vi "USBCam.vi"() -> ()   [LabVIEW 2014]
doc: "This is the main user interface of the Raman spectroscopy system."
uses:
  TypeDef/States.ctl
  <vilib>/Utility/miscctls.llb/LVPoint32TypeDef.ctl
  TypeDef/LaserSpot.ctl
panel:
  out "Spot Y":dbl
  out "Spot X":dbl
  in  "Box":cluster{"Width":dbl, " Height":dbl}={"Width"=200.0, " Height"=214.0}
  in  "Down":bool
  in  "Top":bool
  in  "Right":bool
  in  "Left":bool
  in  "Snap":bool
  out "Boolean":bool
  in  "LaserSpot":bool
  out "Initialization finished":bool
  out "ZoomRatio":dbl format="%#_2g"
  out "Live video":picture caption="600 x 480"
  in  "Camera ID":u32
  out "Bits/Pixel":i32=8
  in  "Autogain":bool
  in  "Master Gain":i32(slide) min=0 max=100 scale=0.0..100.0
  in  "Hotpixel correction 2":bool
  in  "Blacklevel compensation":bool
  in  "Edge Filter":i32(ring)=2 items=["High"=1, "Low"=2]
  in  "Edge Filter Enable / Disable":bool
  in  "Exposure time (ms)":dbl(slide)=100.65900000000002 min=0.06675 max=71.556 step=0.06675 scale=0.06675..71.556 scale format="%#.3g"
  in  "Pixel clock":i32(slide)=20 min=5 max=43 scale=5.0..43.0
  in  "Frame rate":dbl(slide)=9.827169720568149 min=4.876716604244694 max=13.962044182888818 step=6.675e-05 scale=4.876716604244694..13.962044182888818 scale format="%^#_3g"
  in  "Blacklevel Offset":i32(slide) min=0 max=255 scale=0.0..255.0
  out "FPS":dbl=6.258409738085552
  out "Width":i32=640
  out "Height":i32=480
  in  "Quit":bool
  # "Camera Control"
  # "Objective: CFI Plan Fluor ELWD 60x (1.27 NA) \nThe depth of field: 1.78 um\nPixel Size: 0.0877um/px"
  # "Adjust laser spot lightly"
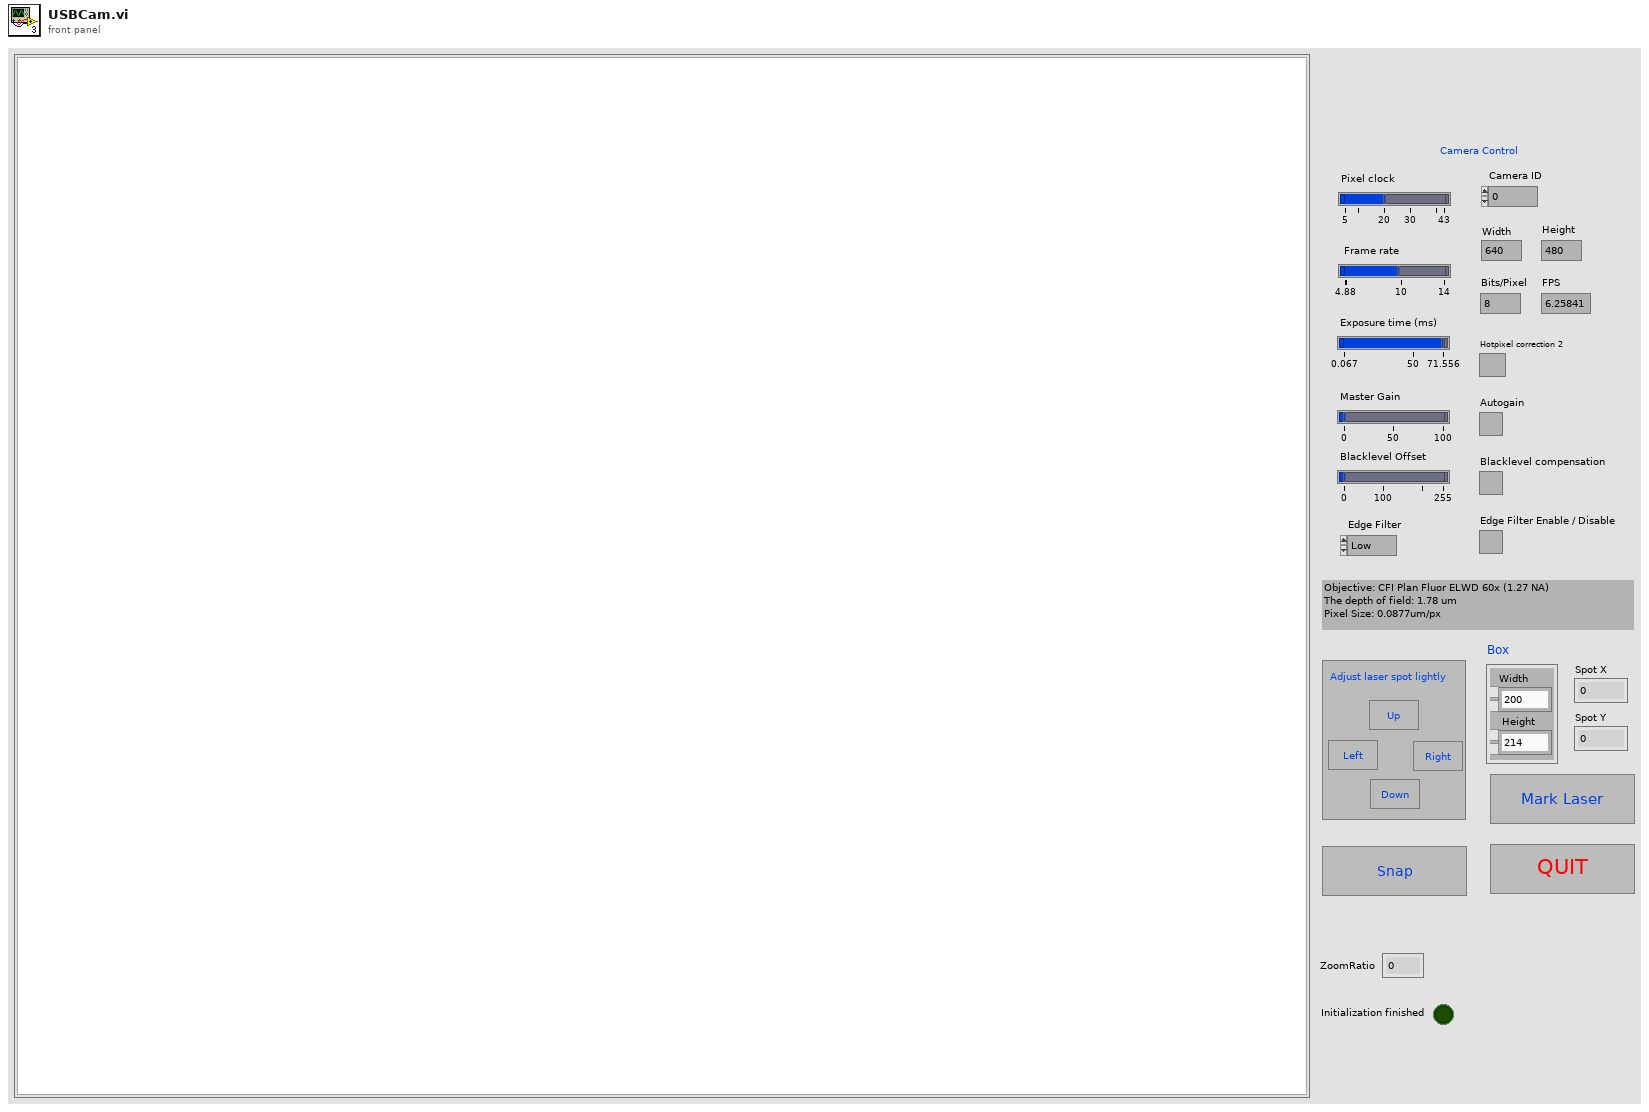
[diagram p1: front panel]
types:
  T1 = typedef "LaserSpot.ctl" = cluster{"Laser X":dbl, "Laser Y":dbl}
  T2 = cluster{"left":i16, "top":i16, "right":i16, "bottom":i16}
  T3 = typedef "LVPoint32TypeDef.ctl" = cluster{"Horizontal":i32, "Vertical":i32}
  T4 = typedef "States.ctl" = enum16{"Initialize", "CMOS live", "Shut down"}
  T5 = cluster{"Width":u16, "Style":enum32{"Solid", "Dash", "Dot", "DashDot", "DashDotDot"}}
  T6 = typedef "LVBoundsTypeDef.ctl" = cluster{"Width":u32, "Height":u32}
  T7 = typedef "imagedata.ctl" = cluster{"image type":i32, "image depth":i32, "image":u8[], "mask":u8[], "colors":u32[], "Rectangle":cluster{"left":i16, "top":i16, "right":i16, "bottom":i16}}
  T8 = typedef "LVPositionTypeDef.ctl" = cluster{"Left":i32, "Top":i32}
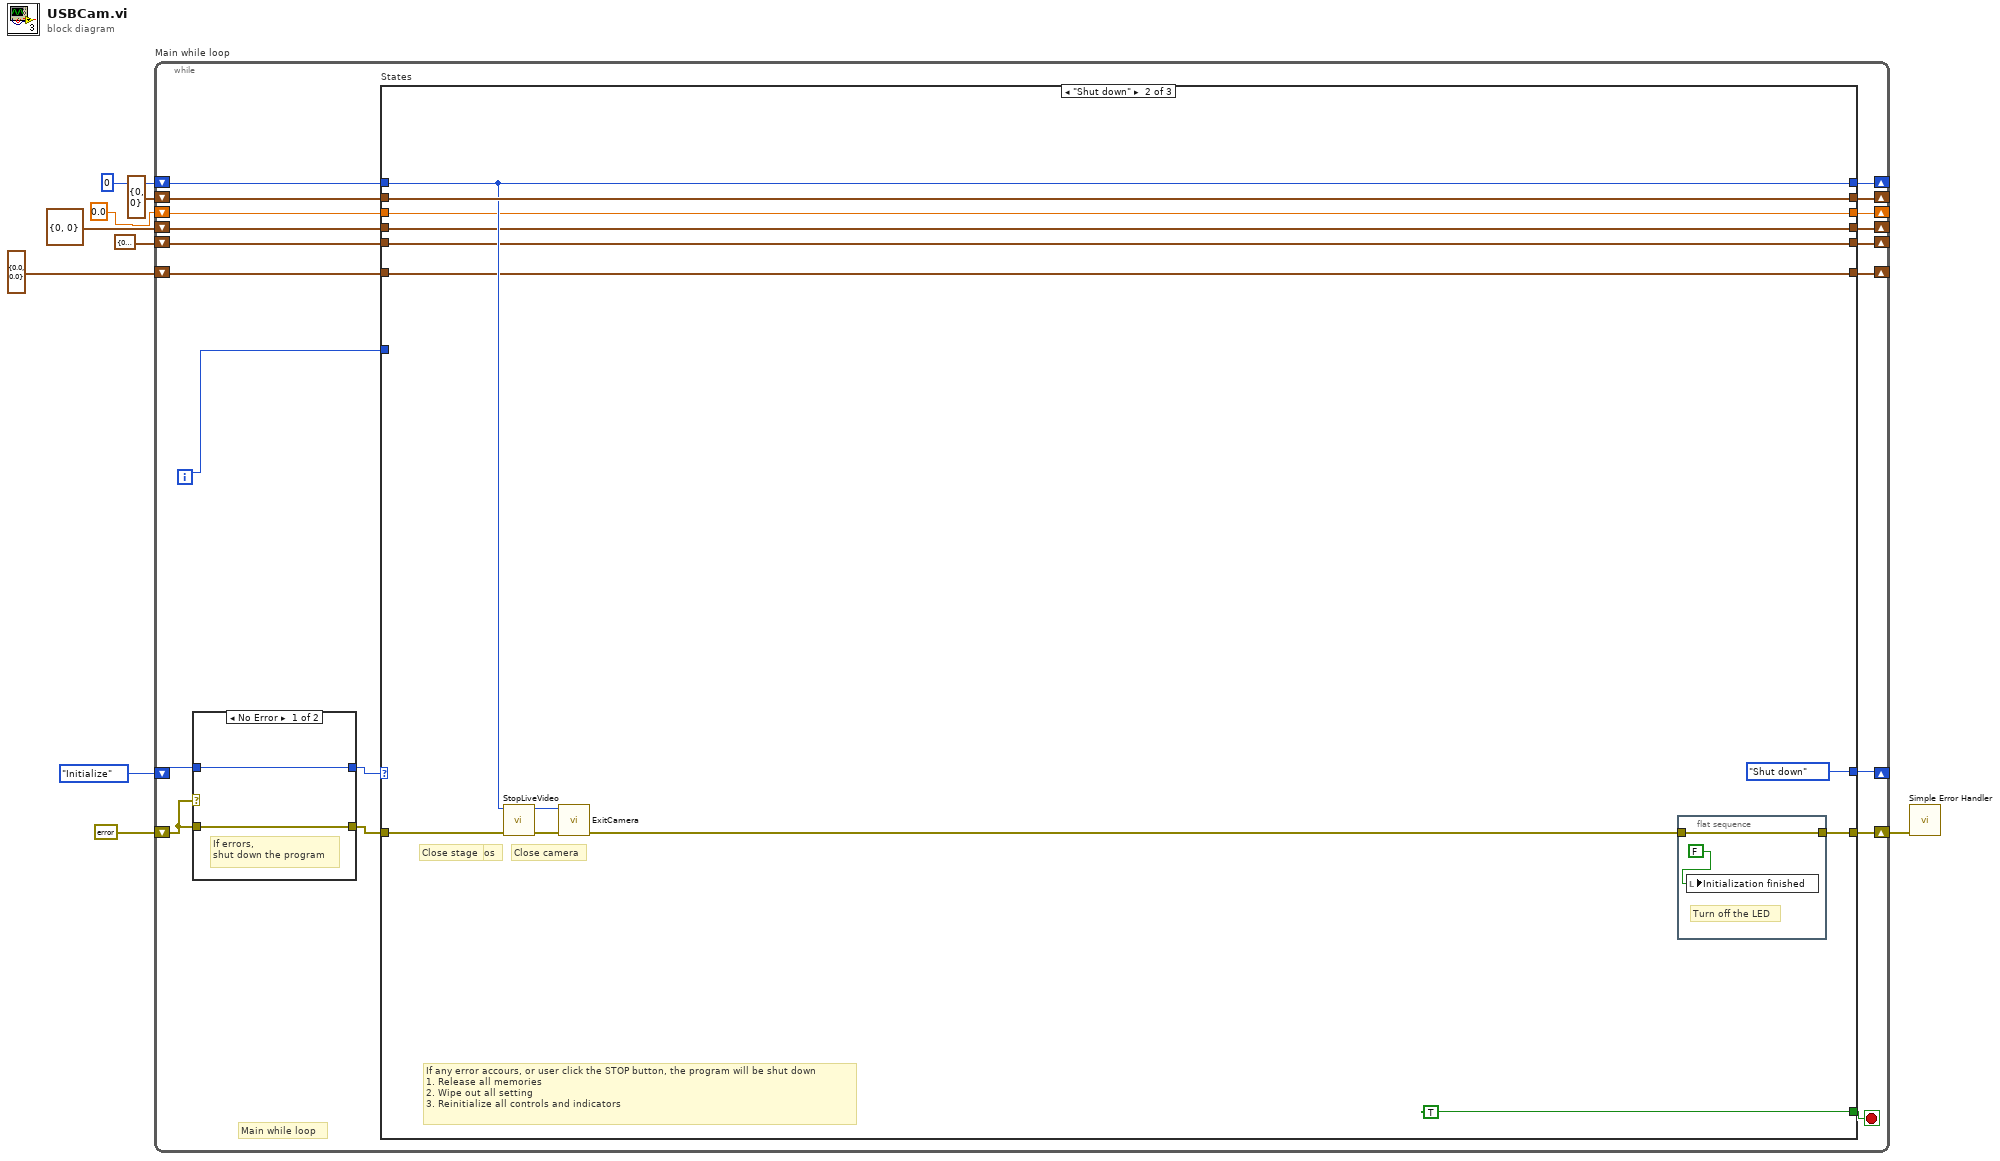
[diagram p0: block diagram]
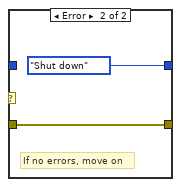
[diagram p2: hidden frame]
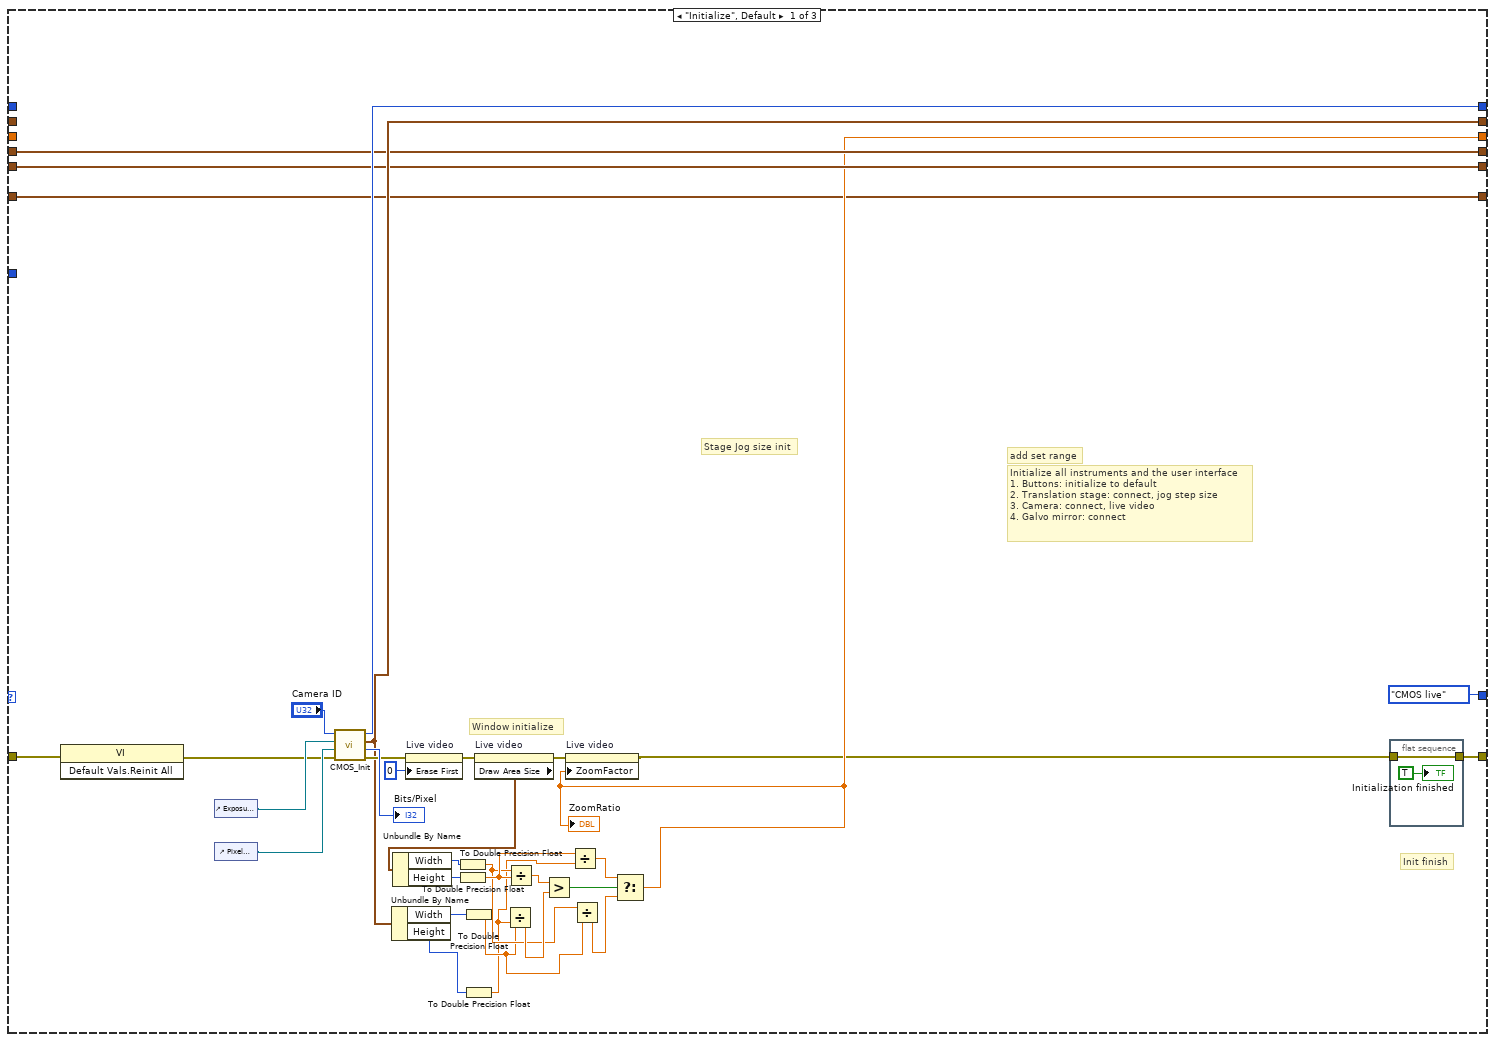
[diagram p3: hidden frame]
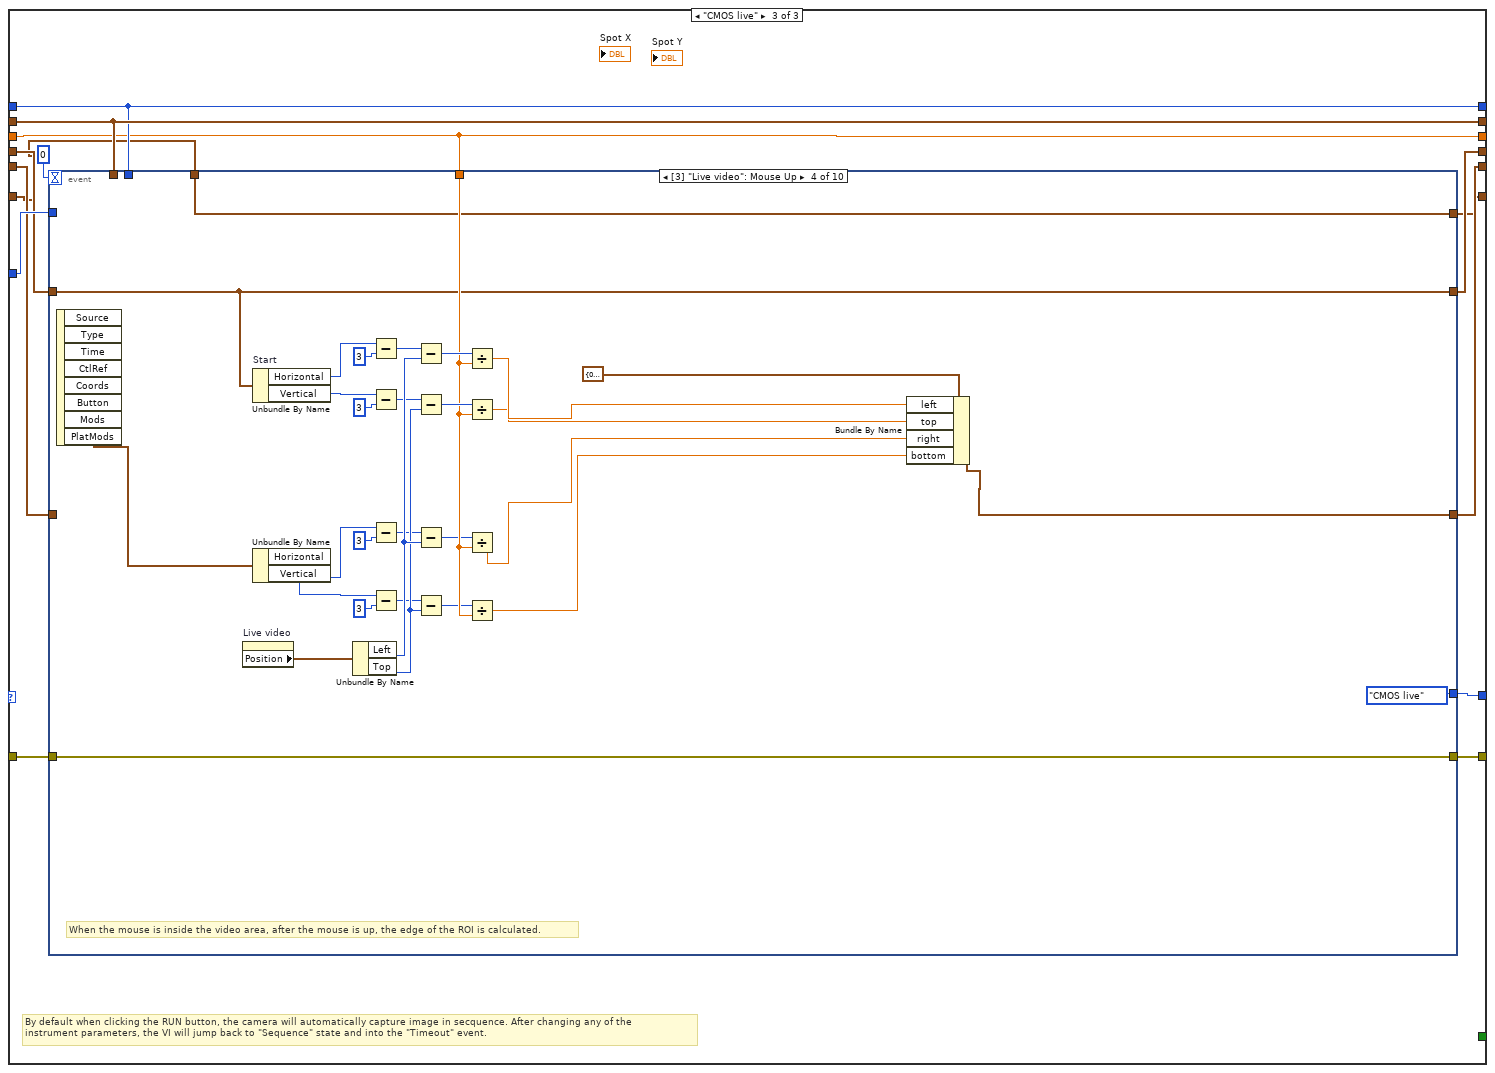
[diagram p4: hidden frame]
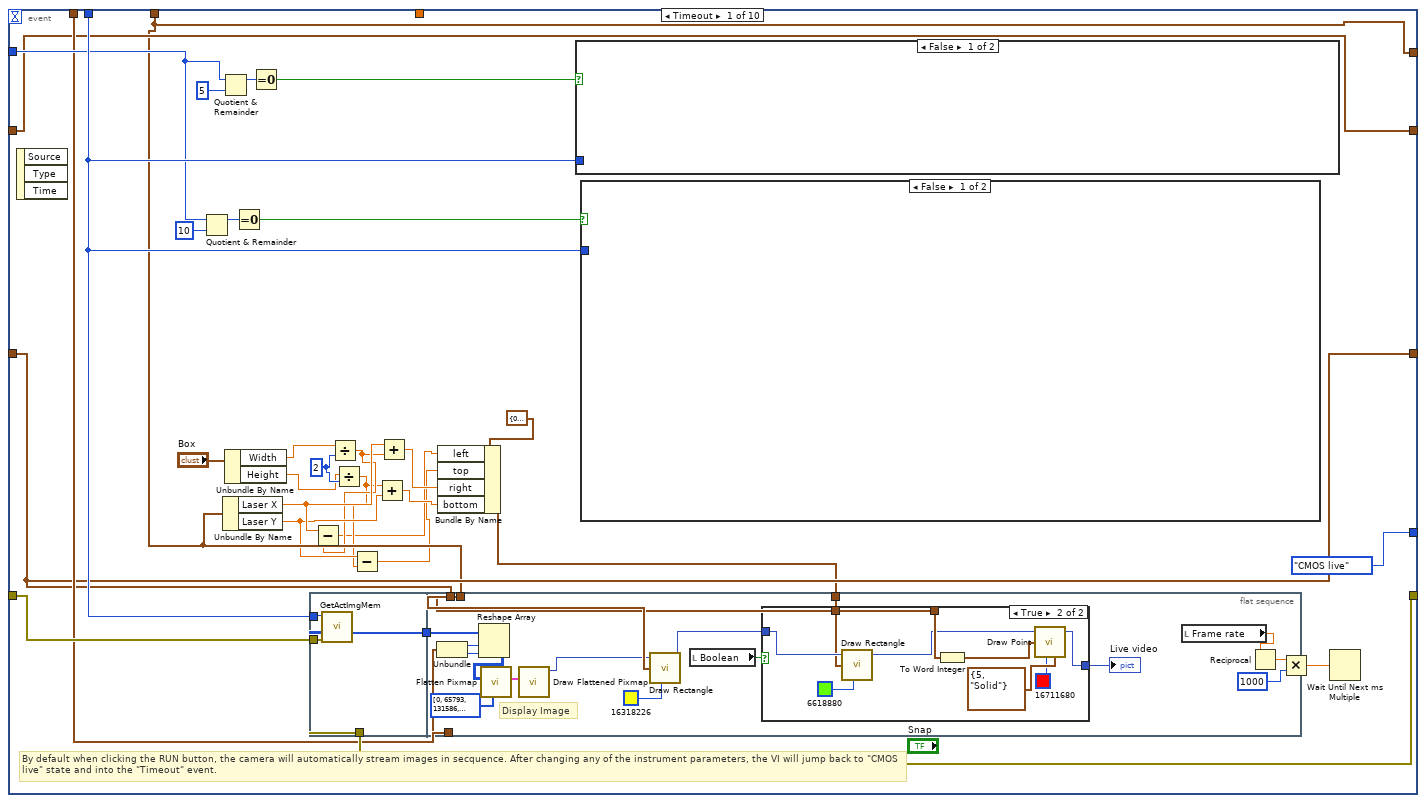
[diagram p5: hidden frame]
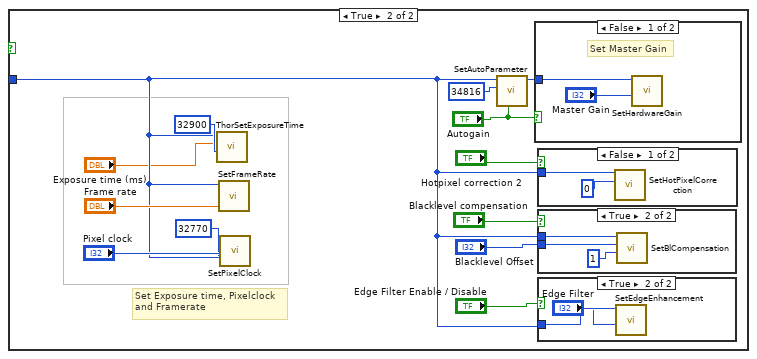
[diagram p6: hidden frame]
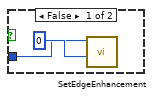
[diagram p7: hidden frame]
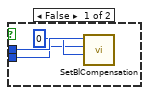
[diagram p8: hidden frame]
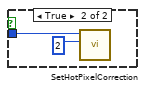
[diagram p9: hidden frame]
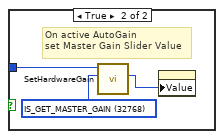
[diagram p10: hidden frame]
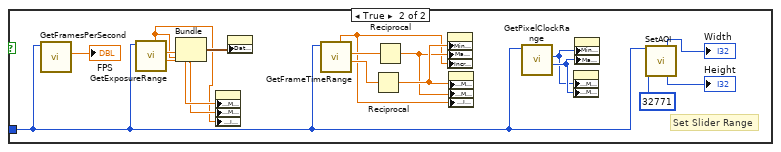
[diagram p11: hidden frame]
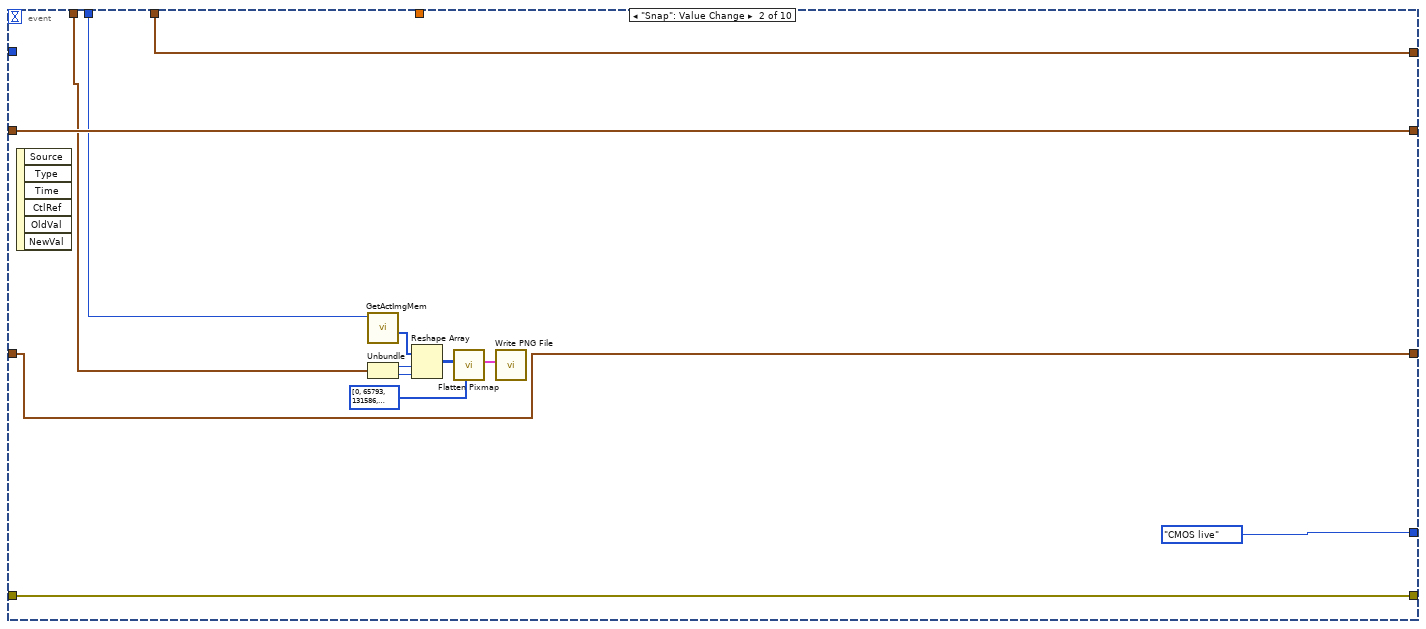
[diagram p13: hidden frame]
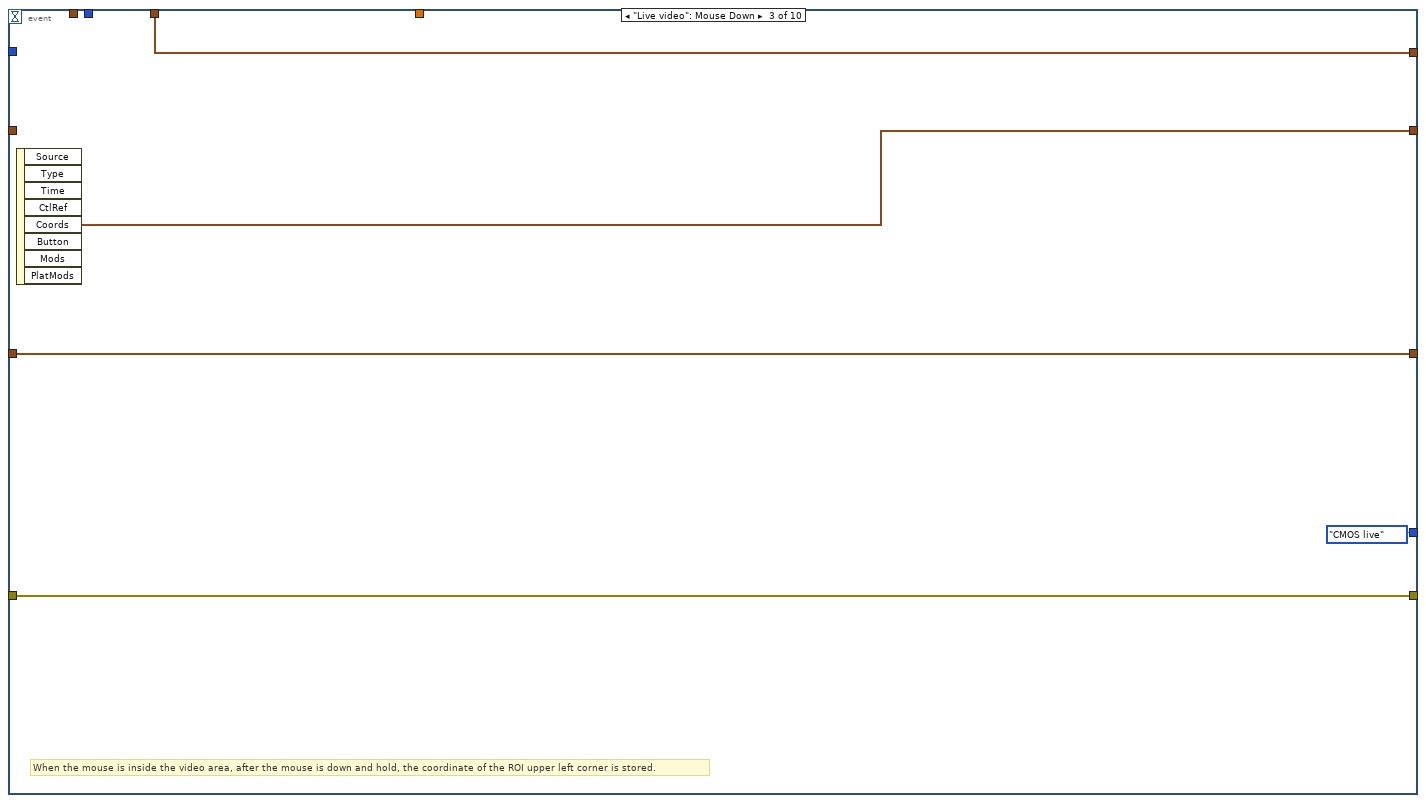
[diagram p14: hidden frame]
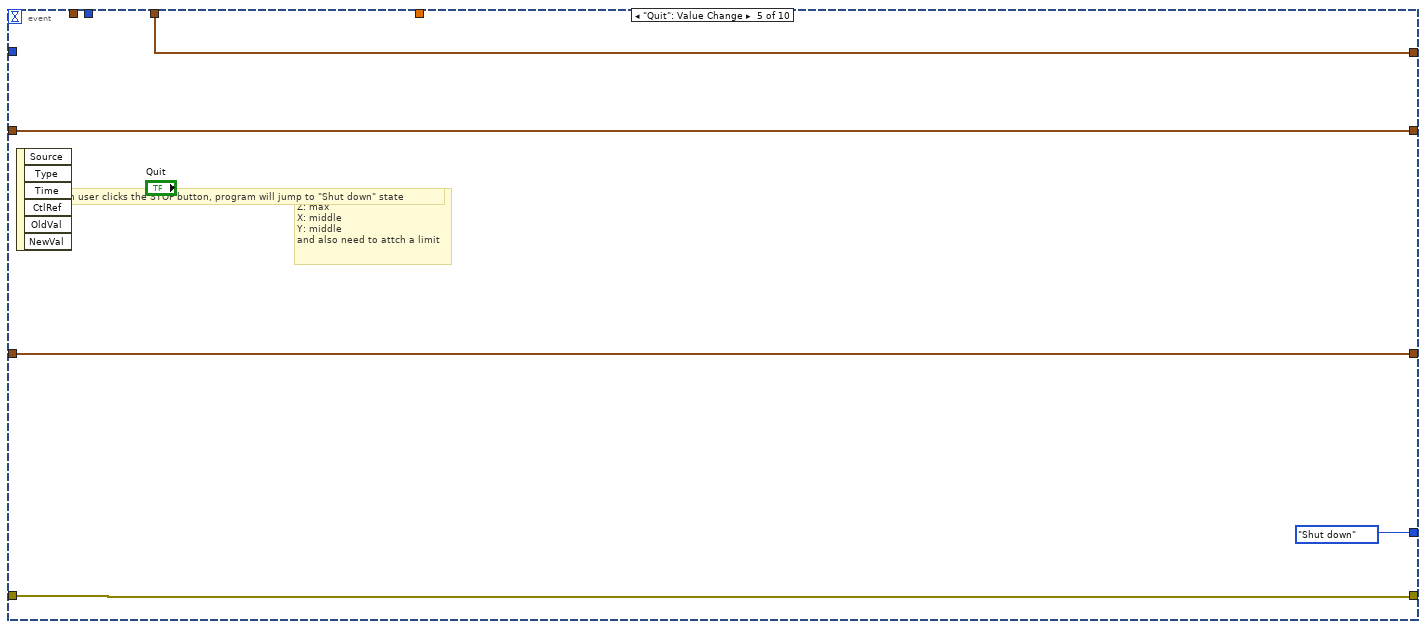
[diagram p15: hidden frame]
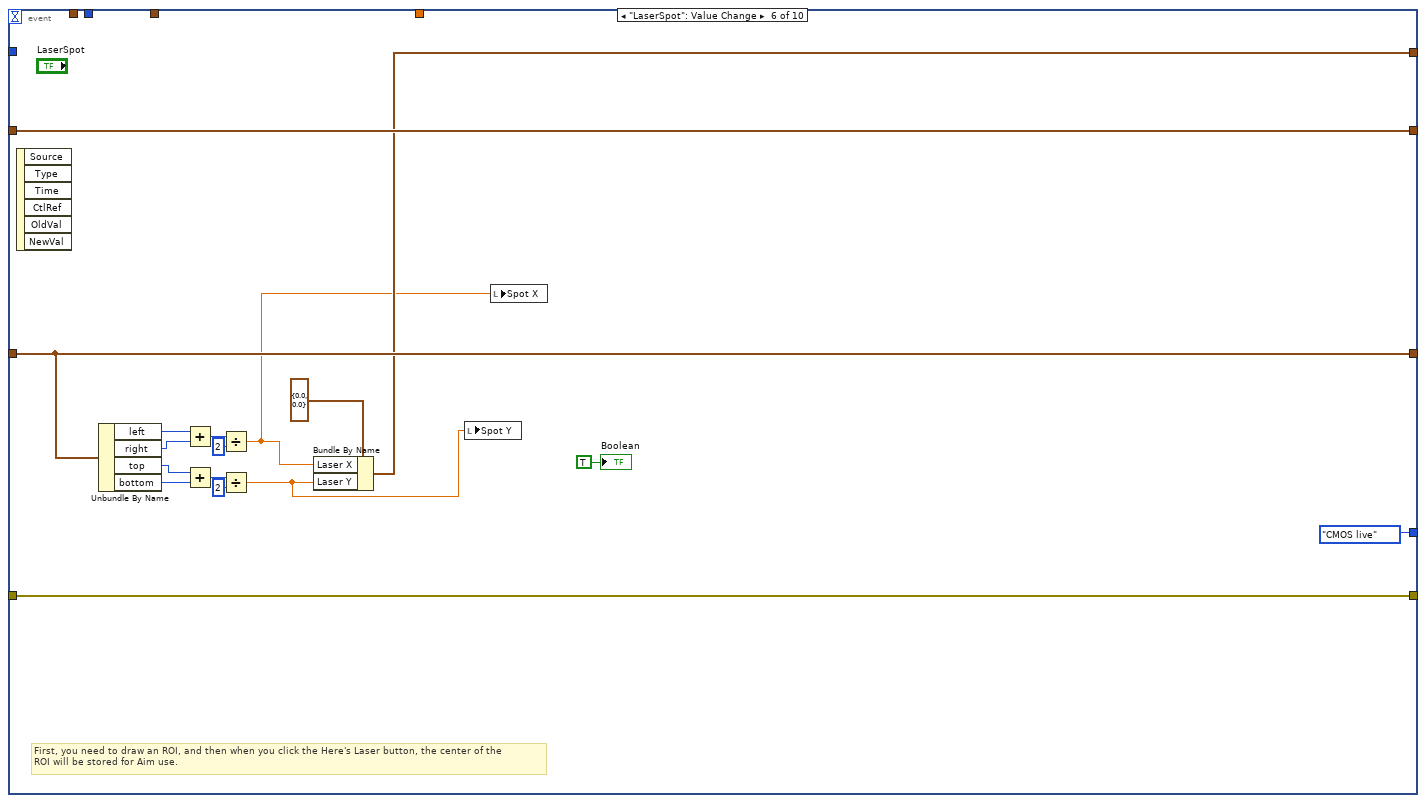
[diagram p16: hidden frame]
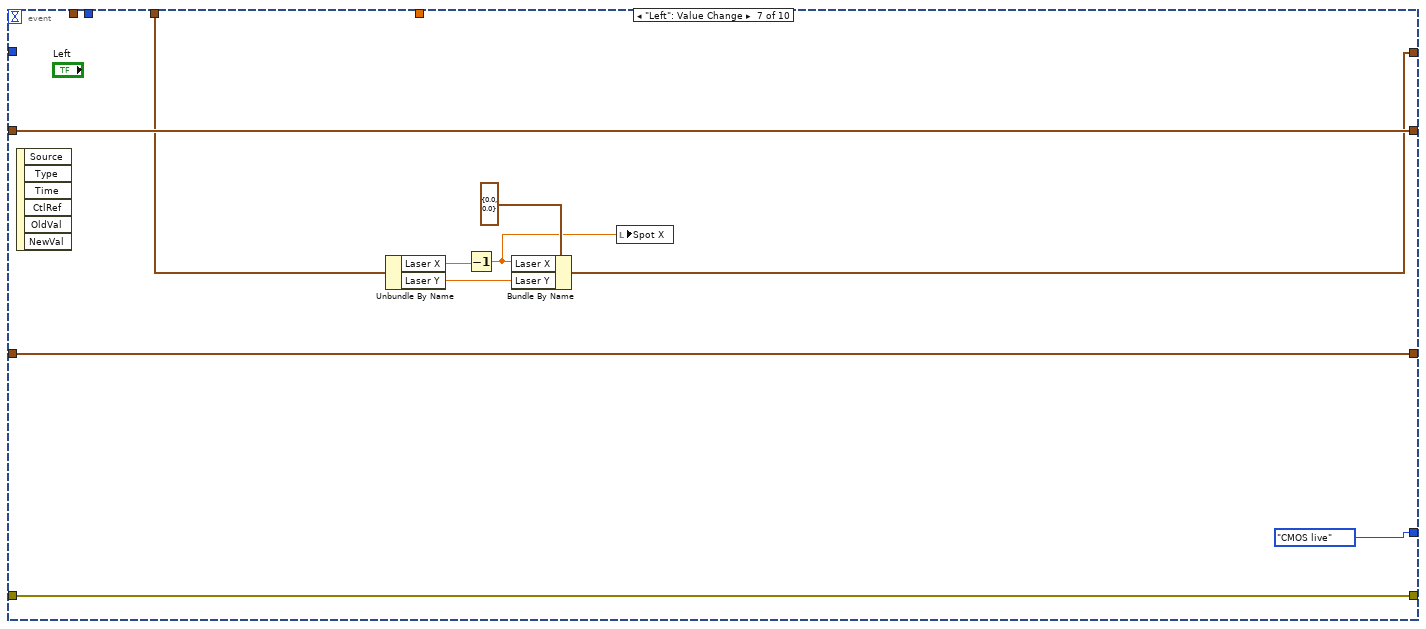
[diagram p17: hidden frame]
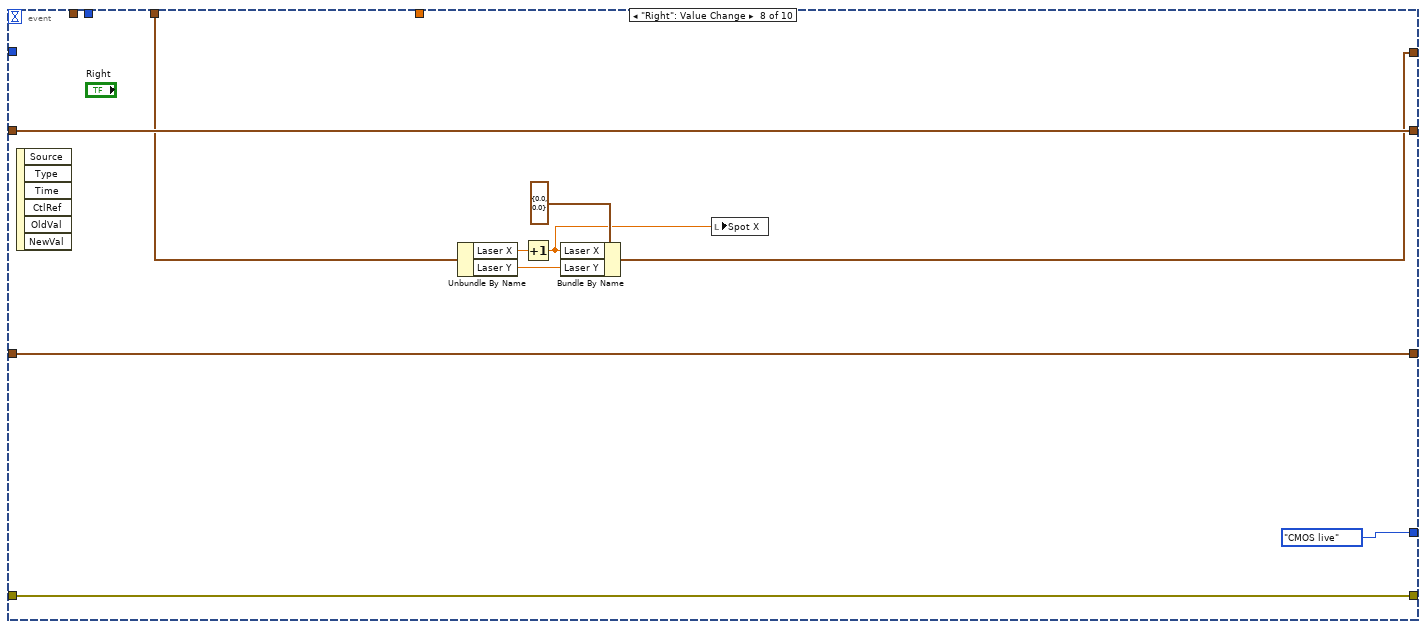
[diagram p18: hidden frame]
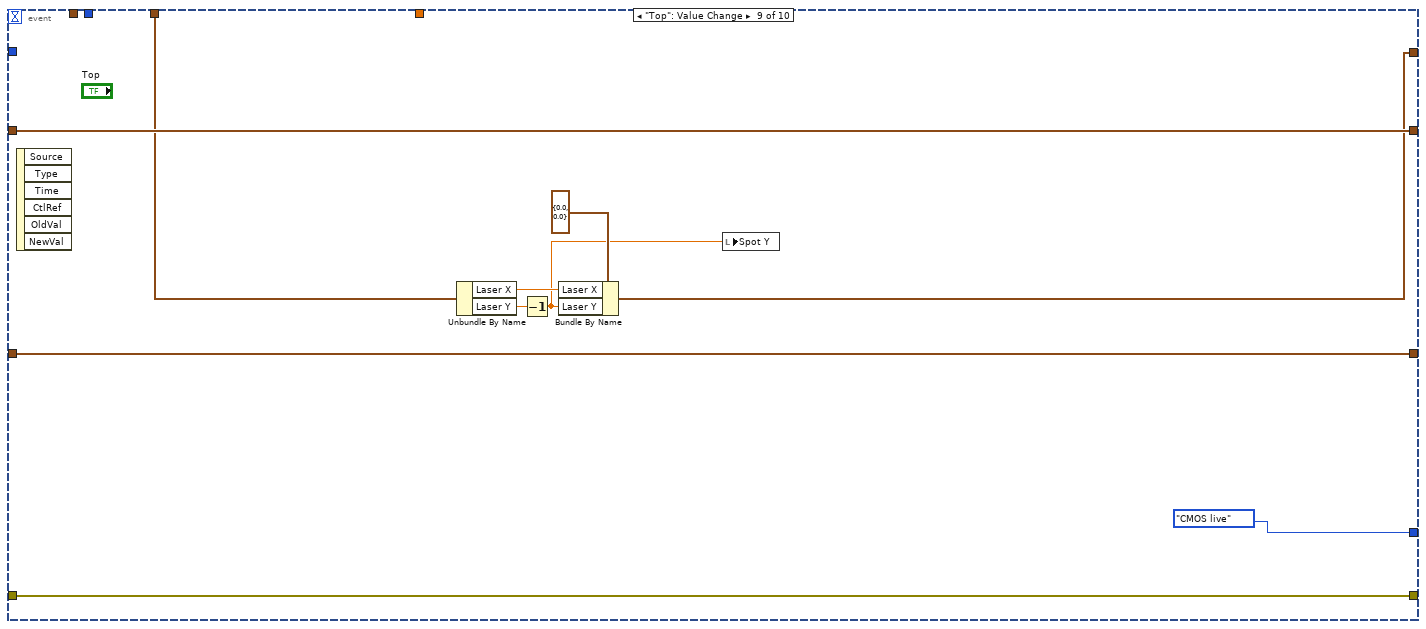
[diagram p19: hidden frame]
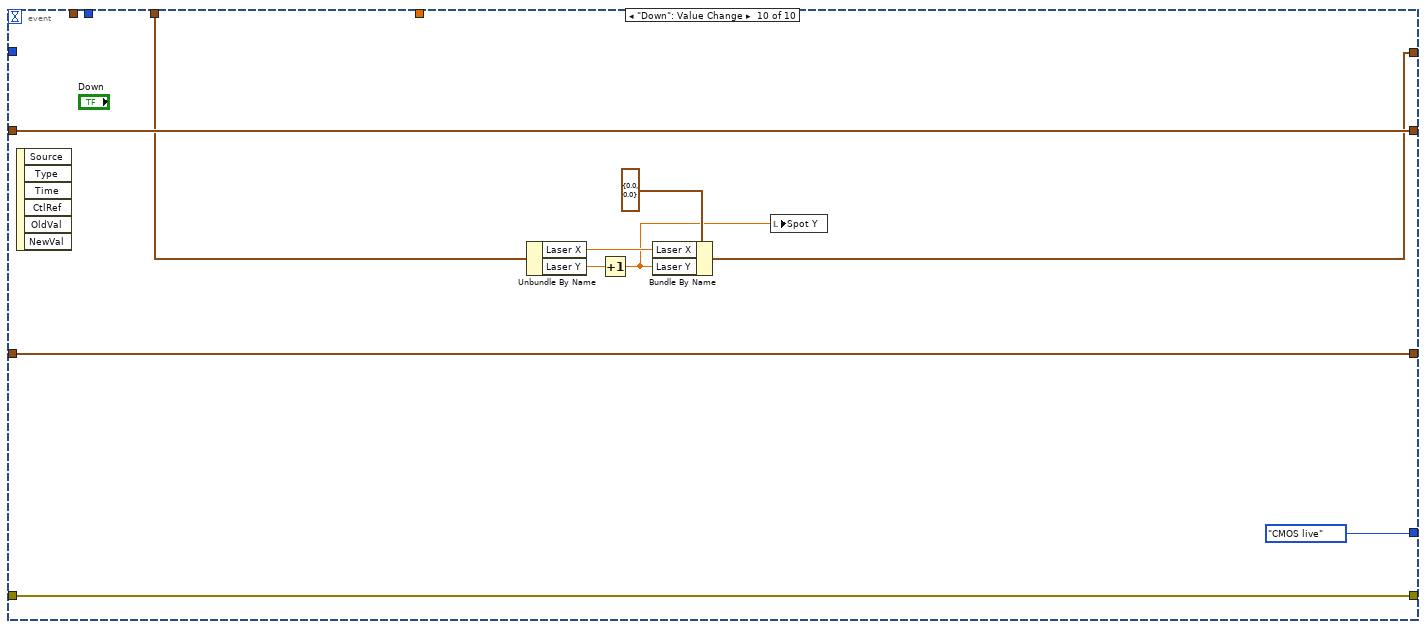
[diagram p20: hidden frame]
diagram:
  n1 = while "Main while loop" {
    shift-right: [w24] -> _
    shift-left: States."Initialize" -> [w29]
    shift-right: [w27] -> w7
    shift-left: errorcluster {"status"=FALSE, "code"=0, "source"=""} ("error out") -> [w23]
    shift-right: [w22] -> _
    shift-left: u32 0 ("CMOS Handle Out") -> [w21]
    shift-right: [w19] -> _
    shift-left: cluster{"Height":i32, "Width":i32} {"Height"=0, "Width"=0} ("WidthAndHeight") -> [w18]
    shift-right: [w17] -> _
    shift-left: 0.0 -> [w12]
    shift-right: [w16] -> _
    shift-left: T3 {"Horizontal"=0, "Vertical"=0} ("Coords") -> [w15]
    shift-right: [w14] -> _
    shift-left: T2 {"left"=0, "top"=0, "right"=0, "bottom"=0} ("rect") -> [w13]
    shift-right: [w11] -> _
    shift-left: T1 {"Laser X"=0.0, "Laser Y"=0.0} ("LaserSpot 2") -> [w10]
    i -> [w20]
    stop <- w25 stop-if-true
    # "Main while loop"
    n2 = case shown="No Error" w23 {
      tunnel: w23 -> [w31 w33]
      tunnel: [w31 w33] -> w26
      tunnel: w29 -> [w30 _]
      tunnel: [w30 States."Shut down"] -> w28
      frame No Error {
        # "If errors,\nshut down the program"
      }
      frame Error {
        # "If no errors, move on"
      }
    }
    n3 = case "States" shown="\"Shut down\"" w28 {
      tunnel: [w35 w72 w95] -> w27
      tunnel: w26 -> [w65 w69 w96]
      tunnel: [_ TRUE _] -> w25
      tunnel: [States."CMOS live" States."Shut down" w97] -> w24
      tunnel: [w64 w76 w91] -> w22
      tunnel: w21 -> [_ w76 w91]
      tunnel: w20 -> [_ _ w93]
      tunnel: [w45 w79 w92] -> w19
      tunnel: w18 -> [_ w79 w92]
      tunnel: [w38 w75 w86] -> w17
      tunnel: w12 -> [_ w75 w86]
      tunnel: [w40 w74 w90] -> w16
      tunnel: w15 -> [w40 w74 w89]
      tunnel: [w39 w73 w88] -> w14
      tunnel: w13 -> [w39 w73 w87]
      tunnel: [w37 w71 w85] -> w11
      tunnel: w10 -> [w37 w71 w84]
      frame "Initialize", Default {
        # "Init finish"
        # "add set range"
        # "Stage Jog size init"
        # "Window initialize"
        # "Initialize all instruments and the user interface\n1. Buttons: initialize to default\n2. Translation stage: connect, jog step size\n3. Camera: connect, live video\n4. Galvo mirror: connect"
        n4 = invoke class="VI" method="Default Vals.Reinit All"(error in=w65) -> (error out=w36:errorcluster)  [unwired: 2 in, 2 out]
        n5 = control-ref of="Exposure time (ms)"() -> (w63:refnum<vi>)
        n6 = control-ref of="Pixel clock"() -> (w62:refnum<vi>)
        n7 = call "CMOS_Init.vi"("error in"=w36, "Pixel clock"=w62, "Exposure time"=w63, "Camera ID"="Camera ID") -> ("error out"=w59:errorcluster, "Bits/Pixel"=→"Bits/Pixel":i32, "WidthAndHeight"=w45:cluster{"Height":i32, "Width":i32}, "CMOS Handle Out"=w64:u32)  [unwired: 3 in]
        n8 = Unbundle By Name(w45) -> ("Width"=w44:i32, "Height"=w43:i32)
        n9 = property on="Live video" class="Pict"(error in=w59, "Erase First"=u8 0) -> (error out=w47:errorcluster)  [unwired: 1 in, 1 out]
        n10 = To Double Precision Float(number=w44) -> (double precision float=w42:dbl)
        n11 = To Double Precision Float(number=w43) -> (double precision float=w41:dbl)
        n12 = property on="Live video" class="Pict"(error in=w47) -> (error out=w46:errorcluster, "Draw Area Size"=w57:T6)  [unwired: 1 in, 1 out]
        n13 = Unbundle By Name(w57) -> ("Width"=w55:u32, "Height"=w56:u32)
        n14 = To Double Precision Float(number=w55) -> (double precision float=w49:dbl)
        n15 = To Double Precision Float(number=w56) -> (double precision float=w51:dbl)
        n16 = Divide(x=w42, y=w41) -> (x/y=w52:dbl)
        n17 = Divide(x=w49, y=w51) -> (x/y=w54:dbl)
        n18 = Greater?(x=w54, y=w52) -> (0:w53:bool)
        n19 = Divide(x=w51, y=w41) -> (x/y=w50:dbl)
        n20 = Divide(x=w49, y=w42) -> (x/y=w48:dbl)
        n21 = Select(t=w50, s=w53, f=w48) -> (s? t:f=w38:dbl)
        "ZoomRatio" <- w38
        n22 = property on="Live video" class="Pict"(error in=w46, "ZoomFactor"=w38) -> (error out=w34:errorcluster)  [unwired: 1 in, 1 out]
        n23 = flat-sequence {
          tunnel: [w67] -> w35
          tunnel: w34 -> [w67]
          frame #0 {
            "Initialization finished" <- TRUE ("Initialization finished")
          }
        }
      }
      frame "Shut down" {
        # "Close 3 galvos"
        # "Close camera"
        # "Close stage"
        # "If any error accours, or user click the STOP button, the program will be shut down\n1. Release all memories\n2. Wipe out all setting\n3. Reinitialize all controls and indicators"
        n24 = call "StopLiveVideo.vi"("error in"=w69, "Camera Handle In"=w76) -> ("error out"=w78:errorcluster, "Camera Handle Out"=w77:u32)  [unwired: 8 in]
        n25 = call "ExitCamera.vi"("error in"=w78, "Camera Handle In"=w77) -> ("error out"=w70:errorcluster)  [unwired: 9 in]
        n26 = flat-sequence {
          tunnel: w70 -> [w83]
          tunnel: [w83] -> w72
          frame #0 {
            # "Turn off the LED"
            n27 = local write "Initialization finished"(FALSE ("Initialization finished")) -> ()
          }
        }
      }
      frame "CMOS live" {
        # "By default when clicking the RUN button, the camera will automatically capture image in secquence. After changing any of the \ninstrument parameters, the VI will jump back to \"Sequence\" state and into the \"Timeout\" event."
        n28 = event shown="[3] \"Live video\": Mouse Up" {
          selector: _ -> [_ _ _ _ _ _ _ _ _ _]
          dyn-events: _ -> [_ _ _ _ _ _ _ _ _ _]
          timeout: 0 -> [_ _ _ _ _ _ _ _ _ _]
          tunnel: [States."CMOS live" States."CMOS live" States."CMOS live" States."CMOS live" States."Shut down" States."CMOS live" States."CMOS live" States."CMOS live" States."CMOS live" States."CMOS live"] -> w97
          tunnel: w96 -> [w120 w209 w223 w230 w261 w279 w289 w299 w309 w319]
          tunnel: [w119 w209 w223 w230 w261 w279 w289 w299 w309 w319] -> w95
          tunnel: w91 -> [w118 w218 _ _ _ _ _ _ _ _]
          tunnel: w93 -> [w117 _ _ _ _ _ _ _ _ _]
          tunnel: w92 -> [w116 w211 _ _ _ _ _ _ _ _]
          tunnel: [w114 w221 w225 w232 w260 w278 w288 w298 w308 w318] -> w90
          tunnel: w89 -> [w114 w221 _ w232 w260 w278 w288 w298 w308 w318]
          tunnel: [w115 w220 w224 w235 w259 w268 w287 w297 w307 w317] -> w88
          tunnel: w87 -> [w115 w220 w224 _ w259 w268 w287 w297 w307 w317]
          tunnel: w86 -> [_ _ _ w234 _ _ _ _ _ _]
          tunnel: [w110 w219 w222 w229 w258 w266 w284 w292 w303 w313] -> w85
          tunnel: w84 -> [w110 w219 w222 w229 w258 _ w283 w293 w304 w314]
          event Timeout {
            w109 = 2
            # "By default when clicking the RUN button, the camera will automatically stream images in secquence. After changing any of the instrument parameters, the VI will jump back to \"CMOS live\" state and into the \"Timeout\" event."
            n29 = event-data() -> ()  [unwired: 1 in, 3 out]
            n30 = Quotient & Remainder(x=w117, y=10) -> (x-y*floor(x/y)=w127:i32)  [unwired: 1 out]
            n31 = Quotient & Remainder(x=w117, y=5) -> (x-y*floor(x/y)=w130:i32)  [unwired: 1 out]
            n32 = Unbundle By Name(w110) -> ("Laser X"=w104:dbl, "Laser Y"=w103:dbl)
            n33 = Unbundle By Name("Box") -> ("Width"=w108:dbl, "Height"=w107:dbl)
            n34 = Equal To 0?(x=w127) -> (x = 0?=w125:bool)
            n35 = Equal To 0?(x=w130) -> (x = 0?=w129:bool)
            n36 = flat-sequence {
              tunnel: [w182] -> w131
              tunnel: w118 -> [w183]
              tunnel: w120 -> [w181]
              tunnel: [w180] -> w119
              tunnel: w131 -> [w198]
              tunnel: w116 -> [w197]
              tunnel: w115 -> [w190]
              tunnel: w110 -> [w186]
              tunnel: w98 -> [w184]
              frame #0 {
                n37 = call "GetActImgMem.vi"("error in"=w181, "Camera Handle In"=w183) -> ("error out"=w180:errorcluster, "Image Memory Out"=w182:u8[])  [unwired: 6 in, 2 out]
              }
              frame #1 {
                # "Display Image"
                n38 = Unbundle(w197) -> ("Height"=w196:i32, "Width"=w195:i32)
                n39 = Reshape Array(w198, w196, w195) -> (w194:u8[][])
                n40 = call <vilib>:"Flatten Pixmap.vi"("colors"=u32[] [0, 65793, 131586, 197379, 263172, 328965, 394758, 460551, 526344, 592137, 657930, 723723, 789516, 855309, 921102, 986895, 1052688, 1118481, 1184274, 1250067, 1315860, 1381653, 1447446, 1513239, 1579032, 1644825, 1710618, 1776411, 1842204, 1907997, 1973790, 2039583, 2105376, 2171169, 2236962, 2302755, 2368548, 2434341, 2500134, 2565927, 2631720, 2697513, 2763306, 2829099, 2894892, 2960685, 3026478, 3092271, 3158064, 3223857, 3289650, 3355443, 3421236, 3487029, 3552822, 3618615, 3684408, 3750201, 3815994, 3881787, 3947580, 4013373, 4079166, 4144959, 4210752, 4276545, 4342338, 4408131, 4473924, 4539717, 4605510, 4671303, 4737096, 4802889, 4868682, 4934475, 5000268, 5066061, 5131854, 5197647, 5263440, 5329233, 5395026, 5460819, 5526612, 5592405, 5658198, 5723991, 5789784, 5855577, 5921370, 5987163, 6052956, 6118749, 6184542, 6250335, 6316128, 6381921, 6447714, 6513507, 6579300, 6645093, 6710886, 6776679, 6842472, 6908265, 6974058, 7039851, 7105644, 7171437, 7237230, 7303023, 7368816, 7434609, 7500402, 7566195, 7631988, 7697781, 7763574, 7829367, 7895160, 7960953, 8026746, 8092539, 8158332, 8224125, 8289918, 8355711, 8421504, 8487297, 8553090, 8618883, 8684676, 8750469, 8816262, 8882055, 8947848, 9013641, 9079434, 9145227, 9211020, 9276813, 9342606, 9408399, 9474192, 9539985, 9605778, 9671571, 9737364, 9803157, 9868950, 9934743, 10000536, 10066329, 10132122, 10197915, 10263708, 10329501, 10395294, 10461087, 10526880, 10592673, 10658466, 10724259, 10790052, 10855845, 10921638, 10987431, 11053224, 11119017, 11184810, 11250603, 11316396, 11382189, 11447982, 11513775, 11579568, 11645361, 11711154, 11776947, 11842740, 11908533, 11974326, 12040119, 12105912, 12171705, 12237498, 12303291, 12369084, 12434877, 12500670, 12566463, 12632256, 12698049, 12763842, 12829635, 12895428, 12961221, 13027014, 13092807, 13158600, 13224393, 13290186, 13355979, 13421772, 13487565, 13553358, 13619151, 13684944, 13750737, 13816530, 13882323, 13948116, 14013909, 14079702, 14145495, 14211288, 14277081, 14342874, 14408667, 14474460, 14540253, 14606046, 14671839, 14737632, 14803425, 14869218, 14935011, 15000804, 15066597, 15132390, 15198183, 15263976, 15329769, 15395562, 15461355, 15527148, 15592941, 15658734, 15724527, 15790320, 15856113, 15921906, 15987699, 16053492, 16119285, 16185078, 16250871, 16316664, 16382457, 16448250, 16514043, 16579836, 16645629, 16711422, 0] ("output array 2"), "8-bit pixmap"=w194) -> ("image data"=w193:T7)  [unwired: 9 in]
                n41 = call <vilib>:"Draw Flattened Pixmap.vi"("image data"=w193) -> ("new picture"=w185:picture)  [unwired: 8 in]
                n42 = call <vilib>:"Draw Rectangle.vi"("picture"=w185, "rect"=w190, "color(black)"=u32 16318226) -> ("new picture"=w189:picture)  [unwired: 6 in]
                n43 = local read "Boolean"() -> (w187:bool)
                n44 = case shown="True" w187 {
                  tunnel: w189 -> [w199 w203]
                  tunnel: [w199 w205] -> w188
                  tunnel: w186 -> [_ w204]
                  tunnel: w184 -> [_ w201]
                  frame False {
                  }
                  frame True {
                    n45 = call <vilib>:"Draw Rectangle.vi"("picture"=w203, "rect"=w201, "color(black)"=u32 6618880) -> ("new picture"=w202:picture)  [unwired: 6 in]
                    n46 = To Word Integer(number=w204) -> (16bit integer=w206:cluster{"Laser X":i16, "Laser Y":i16})
                    n47 = call <vilib>:"Draw Point.vi"("picture"=w202, "point(x,y)"=w206, "color(black)"=u32 16711680, "pen"=T5 {"Width"=5, "Style"=enum."Solid"}) -> ("new picture"=w205:picture)  [unwired: 5 in]
                  }
                }
                "Live video" <- w188
              }
            }
            n48 = Divide(x=w108, y=w109) -> (x/y=w102:dbl)
            n49 = Subtract(x=w104, y=w102) -> (x-y=w100:dbl)
            n50 = Divide(x=w107, y=w109) -> (x/y=w101:dbl)
            n51 = Subtract(x=w103, y=w101) -> (x-y=w99:dbl)
            n52 = Add(x=w101, y=w103) -> (x+y=w105:dbl)
            n53 = Add(x=w104, y=w102) -> (x+y=w106:dbl)
            n54 = Bundle By Name(cluster=T2 {"left"=0, "top"=0, "right"=0, "bottom"=0} ("rect"), "left"=w100, "top"=w99, "right"=w106, "bottom"=w105) -> (w98:T2)
            n55 = case shown="False" w129 {
              tunnel: w118 -> [_ w166]
              frame False {
              }
              frame True {
                # "Set Slider Range"
                n56 = call "GetFramesPerSecond.vi"("Camera Handle In"=w166) -> ("FPS"=→"FPS":dbl)  [unwired: 8 in, 2 out]
                n57 = call "GetExposureRange.vi"("Camera Handle In"=w166) -> ("max"=w176:dbl, "min"=w177:dbl, "intervall"=w175:dbl)  [unwired: 6 in, 2 out]
                n58 = Bundle("min"=w177, "max"=w176, "intervall"=w175) -> (w178:cluster{"min":dbl, "max":dbl, "intervall":dbl})  [unwired: 1 in]
                n59 = property on="Exposure time (ms)" class="Schieberegler (strikt)"("Scale.Minimum"=w177, "Scale.Maximum"=w176, "Scale.Increment"=w175) -> ()  [unwired: 2 in, 2 out]
                n60 = property on="Exposure time (ms)" class="Schieberegler (strikt)"("Data Range"=w178) -> ()  [unwired: 2 in, 2 out]
                n61 = call "GetFrameTimeRange.vi"("Camera Handle In"=w166) -> ("max"=w172:dbl, "min"=w171:dbl, "interval"=w168:dbl)  [unwired: 6 in, 2 out]
                n62 = Reciprocal(x=w172) -> (1/x=w170:dbl)
                n63 = Reciprocal(x=w171) -> (1/x=w169:dbl)
                n64 = property on="Frame rate" class="Schieberegler (strikt)"("Minimum"=w170, "Maximum"=w169, "Increment"=w168) -> ()  [unwired: 2 in, 2 out]
                n65 = property on="Frame rate" class="Schieberegler (strikt)"("Scale.Minimum"=w170, "Scale.Maximum"=w169, "Scale.Increment"=w168) -> ()  [unwired: 2 in, 2 out]
                n66 = call "GetPixelClockRange.vi"("Camera Handle In"=w166) -> ("Max"=w174:i32, "Min"=w173:i32)  [unwired: 7 in, 2 out]
                n67 = property on="Pixel clock" class="Schieberegler (strikt)"("Scale.Minimum"=w173, "Scale.Maximum"=w174) -> ()  [unwired: 2 in, 2 out]
                n68 = property on="Pixel clock" class="Schieberegler (strikt)"("Minimum"=w173, "Maximum"=w174) -> ()  [unwired: 2 in, 2 out]
                n69 = call "SetAOI.vi"("Camera Handle In"=w166, "Mode"=32771) -> ("Width Out"=→"Width":i32, "Height Out"=→"Height":i32)  [unwired: 8 in, 4 out]
              }
            }
            n70 = case shown="False" w125 {
              tunnel: w118 -> [_ w135]
              frame False {
              }
              frame True {
                # "Set Exposure time, Pixelclock\nand Framerate"
                n71 = call "ThorSetExposureTime.vi"("Mode"=u16 32900, "Exposure Time"="Exposure time (ms)", "Camera Handle In"=w135) -> ()  [unwired: 6 in, 3 out]
                n72 = call "SetFrameRate.vi"("FPS"="Frame rate", "Camera Handle In"=w135) -> ()  [unwired: 7 in, 3 out]
                n73 = call "SetPixelClock.vi"("Mode"=32770, "Pixel Clock"="Pixel clock", "Camera Handle In"=w135) -> ()  [unwired: 6 in, 3 out]
                n74 = call "SetAutoParameter.vi"("enable"="Autogain", "Param"=34816, "Camera Handle In"=w135) -> ("Camera Handle Out"=w143:u32)  [unwired: 6 in, 2 out]
                n75 = case shown="False" "Autogain" {
                  tunnel: w143 -> [w159 w162]
                  frame False {
                    # "Set Master Gain"
                    n76 = call "SetHardwareGain.vi"("Master Gain"="Master Gain", "Camera Handle In"=w159) -> ()  [unwired: 7 in, 3 out]
                  }
                  frame True {
                    w161 = 32768 items=["IS_GET_MASTER_GAIN"=32768]
                    # "On active AutoGain\nset Master Gain Slider Value"
                    n77 = call "SetHardwareGain.vi"("Mode"=w161, "Camera Handle In"=w162) -> ("Value"=w163:i32)  [unwired: 7 in, 2 out]
                    n78 = property on="Master Gain" class="Slide (strict)"("Value"=w163) -> ()  [unwired: 2 in, 2 out]
                  }
                }
                n79 = case shown="False" "Hotpixel correction 2" {
                  tunnel: w135 -> [w156 w158]
                  frame False {
                    n80 = call "SetHotPixelCorrection.vi"("Mode"=0, "Camera Handle In"=w156) -> ()  [unwired: 7 in, 3 out]
                  }
                  frame True {
                    n81 = call "SetHotPixelCorrection.vi"("Mode"=2, "Camera Handle In"=w158) -> ()  [unwired: 7 in, 3 out]
                  }
                }
                n82 = case shown="True" "Blacklevel compensation" {
                  tunnel: w135 -> [w151 w154]
                  tunnel: "Blacklevel Offset" -> [w149 w152]
                  frame False {
                    n83 = call "SetBlCompensation.vi"("Mode"=0, "offset"=w149, "Camera Handle In"=w151) -> ()  [unwired: 6 in, 3 out]
                  }
                  frame True {
                    n84 = call "SetBlCompensation.vi"("Mode"=1, "offset"=w152, "Camera Handle In"=w154) -> ()  [unwired: 6 in, 3 out]
                  }
                }
                n85 = case shown="True" "Edge Filter Enable / Disable" {
                  tunnel: w135 -> [w145 w148]
                  frame False {
                    n86 = call "SetEdgeEnhancement.vi"("Mode"=0, "Camera Handle In"=w145) -> ()  [unwired: 8 in, 2 out]
                  }
                  frame True {
                    n87 = call "SetEdgeEnhancement.vi"("Mode"="Edge Filter", "Camera Handle In"=w148) -> ()  [unwired: 8 in, 2 out]
                  }
                }
              }
            }
            n88 = local read "Frame rate"() -> (w124:dbl)
            n89 = Reciprocal(x=w124) -> (1/x=w123:dbl)
            n90 = Multiply(x=w123, y=1000) -> (x*y=w121:dbl)
            n91 = Wait Until Next ms Multiple(millisecond multiple=w121) -> ()  [unwired: 1 out]
          }
          event "Snap": Value Change {
            n92 = event-data() -> ()  [unwired: 1 in, 6 out]
            n93 = call "GetActImgMem.vi"("Camera Handle In"=w218) -> ("Image Memory Out"=w213:u8[])  [unwired: 7 in, 3 out]
            n94 = Unbundle(w211) -> ("Height"=w214:i32, "Width"=w215:i32)
            n95 = Reshape Array(w213, w214, w215) -> (w216:u8[][])
            n96 = call <vilib>:"Flatten Pixmap.vi"("colors"=u32[] [0, 65793, 131586, 197379, 263172, 328965, 394758, 460551, 526344, 592137, 657930, 723723, 789516, 855309, 921102, 986895, 1052688, 1118481, 1184274, 1250067, 1315860, 1381653, 1447446, 1513239, 1579032, 1644825, 1710618, 1776411, 1842204, 1907997, 1973790, 2039583, 2105376, 2171169, 2236962, 2302755, 2368548, 2434341, 2500134, 2565927, 2631720, 2697513, 2763306, 2829099, 2894892, 2960685, 3026478, 3092271, 3158064, 3223857, 3289650, 3355443, 3421236, 3487029, 3552822, 3618615, 3684408, 3750201, 3815994, 3881787, 3947580, 4013373, 4079166, 4144959, 4210752, 4276545, 4342338, 4408131, 4473924, 4539717, 4605510, 4671303, 4737096, 4802889, 4868682, 4934475, 5000268, 5066061, 5131854, 5197647, 5263440, 5329233, 5395026, 5460819, 5526612, 5592405, 5658198, 5723991, 5789784, 5855577, 5921370, 5987163, 6052956, 6118749, 6184542, 6250335, 6316128, 6381921, 6447714, 6513507, 6579300, 6645093, 6710886, 6776679, 6842472, 6908265, 6974058, 7039851, 7105644, 7171437, 7237230, 7303023, 7368816, 7434609, 7500402, 7566195, 7631988, 7697781, 7763574, 7829367, 7895160, 7960953, 8026746, 8092539, 8158332, 8224125, 8289918, 8355711, 8421504, 8487297, 8553090, 8618883, 8684676, 8750469, 8816262, 8882055, 8947848, 9013641, 9079434, 9145227, 9211020, 9276813, 9342606, 9408399, 9474192, 9539985, 9605778, 9671571, 9737364, 9803157, 9868950, 9934743, 10000536, 10066329, 10132122, 10197915, 10263708, 10329501, 10395294, 10461087, 10526880, 10592673, 10658466, 10724259, 10790052, 10855845, 10921638, 10987431, 11053224, 11119017, 11184810, 11250603, 11316396, 11382189, 11447982, 11513775, 11579568, 11645361, 11711154, 11776947, 11842740, 11908533, 11974326, 12040119, 12105912, 12171705, 12237498, 12303291, 12369084, 12434877, 12500670, 12566463, 12632256, 12698049, 12763842, 12829635, 12895428, 12961221, 13027014, 13092807, 13158600, 13224393, 13290186, 13355979, 13421772, 13487565, 13553358, 13619151, 13684944, 13750737, 13816530, 13882323, 13948116, 14013909, 14079702, 14145495, 14211288, 14277081, 14342874, 14408667, 14474460, 14540253, 14606046, 14671839, 14737632, 14803425, 14869218, 14935011, 15000804, 15066597, 15132390, 15198183, 15263976, 15329769, 15395562, 15461355, 15527148, 15592941, 15658734, 15724527, 15790320, 15856113, 15921906, 15987699, 16053492, 16119285, 16185078, 16250871, 16316664, 16382457, 16448250, 16514043, 16579836, 16645629, 16711422, 0] ("output array 2"), "8-bit pixmap"=w216) -> ("image data"=w210:T7)  [unwired: 9 in]
            n97 = call <vilib>:"Write PNG File.vi"("image data"=w210) -> ()  [unwired: 9 in, 2 out]
          }
          event "Live video": Mouse Down {
            # "When the mouse is inside the video area, after the mouse is down and hold, the coordinate of the ROI upper left corner is stored."
            n98 = event-data() -> ("Coords"=w225:T3)  [unwired: 1 in, 7 out]
          }
          event "Live video": Mouse Up {
            # "When the mouse is inside the video area, after the mouse is up, the edge of the ROI is calculated."
            n99 = event-data() -> ("Coords"=w233:T3)  [unwired: 1 in, 7 out]
            n100 = property on="Live video" class="Pict"() -> ("Position"=w231:T8)  [unwired: 2 in, 2 out]
            n101 = Unbundle By Name "Start"(w232) -> ("Horizontal"=w253:i32, "Vertical"=w250:i32)
            n102 = Unbundle By Name(w233) -> ("Horizontal"=w247:i32, "Vertical"=w244:i32)
            n103 = Unbundle By Name(w231) -> ("Left"=w255:i32, "Top"=w254:i32)
            n104 = Subtract(x=w253, y=3) -> (x-y=w251:i32)
            n105 = Subtract(x=w250, y=3) -> (x-y=w249:i32)
            n106 = Subtract(x=w247, y=3) -> (x-y=w245:i32)
            n107 = Subtract(x=w244, y=3) -> (x-y=w242:i32)
            n108 = Subtract(x=w251, y=w255) -> (x-y=w241:i32)
            n109 = Subtract(x=w249, y=w254) -> (x-y=w240:i32)
            n110 = Subtract(x=w245, y=w255) -> (x-y=w228:i32)
            n111 = Subtract(x=w242, y=w254) -> (x-y=w227:i32)
            n112 = Divide(x=w241, y=w234) -> (x/y=w239:dbl)
            n113 = Divide(x=w240, y=w234) -> (x/y=w238:dbl)
            n114 = Divide(x=w228, y=w234) -> (x/y=w237:dbl)
            n115 = Divide(x=w227, y=w234) -> (x/y=w236:dbl)
            n116 = Bundle By Name(cluster=T2 {"left"=0, "top"=0, "right"=0, "bottom"=0} ("rect"), "left"=w239, "top"=w238, "right"=w237, "bottom"=w236) -> (w235:T2)
          }
          event "Quit": Value Change {
            # "Add recover initial position\nZ: max\nX: middle\nY: middle\nand also need to attch a limit"
            # "When user clicks the STOP button, program will jump to \"Shut down\" state"
            n117 = event-data() -> ()  [unwired: 1 in, 6 out]
          }
          event "LaserSpot": Value Change {
            # "First, you need to draw an ROI, and then when you click the Here's Laser button, the center of the\nROI will be stored for Aim use."
            n118 = event-data() -> ()  [unwired: 1 in, 6 out]
            n119 = Unbundle By Name(w268) -> ("left"=w275:i16, "right"=w276:i16, "top"=w270:i16, "bottom"=w269:i16)
            n120 = Add(x=w275, y=w276) -> (x+y=w274:i16)
            n121 = Add(x=w270, y=w269) -> (x+y=w271:i16)
            n122 = Divide(x=w274, y=i16 2) -> (x/y=w264:dbl)
            n123 = Divide(x=w271, y=i16 2) -> (x/y=w263:dbl)
            n124 = Bundle By Name(cluster=T1 {"Laser X"=0.0, "Laser Y"=0.0} ("LaserSpot"), "Laser X"=w264, "Laser Y"=w263) -> (w266:T1)
            n125 = local write "Spot Y"(w263) -> ()
            n126 = local write "Spot X"(w264) -> ()
            "Boolean" <- TRUE ("Boolean")
          }
          event "Left": Value Change {
            n127 = event-data() -> ()  [unwired: 1 in, 6 out]
            n128 = Unbundle By Name(w283) -> ("Laser X"=w281:dbl, "Laser Y"=w282:dbl)
            n129 = Decrement(x=w281) -> (x-1=w280:dbl)
            n130 = Bundle By Name(cluster=T1 {"Laser X"=0.0, "Laser Y"=0.0} ("LaserSpot"), "Laser X"=w280, "Laser Y"=w282) -> (w284:T1)
            n131 = local write "Spot X"(w280) -> ()
          }
          event "Right": Value Change {
            n132 = event-data() -> ()  [unwired: 1 in, 6 out]
            n133 = Unbundle By Name(w293) -> ("Laser X"=w291:dbl, "Laser Y"=w294:dbl)
            n134 = Increment(x=w291) -> (x+1=w290:dbl)
            n135 = Bundle By Name(cluster=T1 {"Laser X"=0.0, "Laser Y"=0.0} ("LaserSpot"), "Laser X"=w290, "Laser Y"=w294) -> (w292:T1)
            n136 = local write "Spot X"(w290) -> ()
          }
          event "Top": Value Change {
            n137 = event-data() -> ()  [unwired: 1 in, 6 out]
            n138 = Unbundle By Name(w304) -> ("Laser X"=w302:dbl, "Laser Y"=w301:dbl)
            n139 = Decrement(x=w301) -> (x-1=w300:dbl)
            n140 = Bundle By Name(cluster=T1 {"Laser X"=0.0, "Laser Y"=0.0} ("LaserSpot"), "Laser X"=w302, "Laser Y"=w300) -> (w303:T1)
            n141 = local write "Spot Y"(w300) -> ()
          }
          event "Down": Value Change {
            n142 = event-data() -> ()  [unwired: 1 in, 6 out]
            n143 = Unbundle By Name(w314) -> ("Laser X"=w312:dbl, "Laser Y"=w311:dbl)
            n144 = Increment(x=w311) -> (x+1=w310:dbl)
            n145 = Bundle By Name(cluster=T1 {"Laser X"=0.0, "Laser Y"=0.0} ("LaserSpot"), "Laser X"=w312, "Laser Y"=w310) -> (w313:T1)
            n146 = local write "Spot Y"(w310) -> ()
          }
        }
      }
    }
  }
  n147 = call <vilib>:"Simple Error Handler.vi"("error in (no error)"=w7) -> ()  [unwired: 4 in, 5 out]
